vi "Check if good target.vi"(6 "Avg Factor":i32, 7 "Limits":T1, 8 "y2-R":dbl, 9 "x2-R":dbl, 10 "y1-L":dbl, 11 "x1-L":dbl) -> (0 "y2 (R) out":dbl, 1 "x2 (L) out":dbl, 2 "y1 (L) out":dbl, 3 "x1 (L) out":dbl, 5 "Good target?":bool)   [LabVIEW 2018]
uses:
  <vilib>/ptbypt/NI_PtbyPt.lvlib
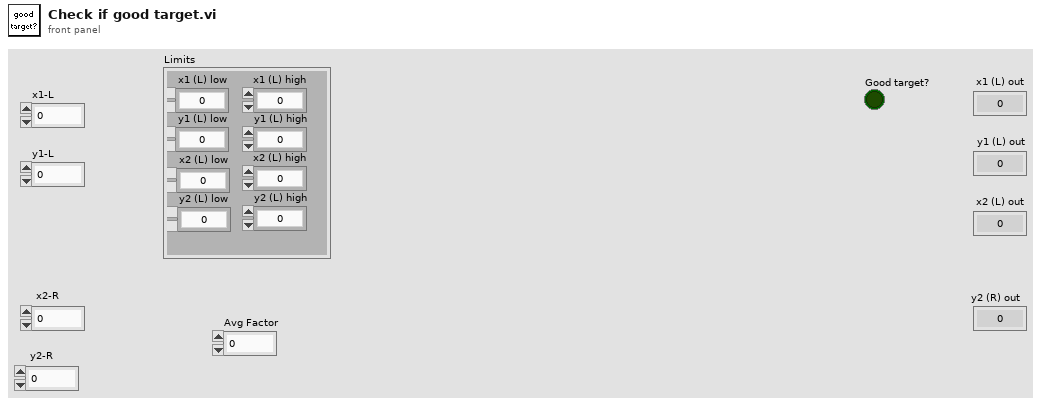
[diagram p1: front panel]
types:
  T1 = cluster{"x1 (L) low":dbl, "x1 (L) high":dbl, "y1 (L) low ":dbl, "y1 (L) high":dbl, "x2 (L) low":dbl, "x2 (L) high":dbl, "y2 (L) low":dbl, "y2 (L) high":dbl}
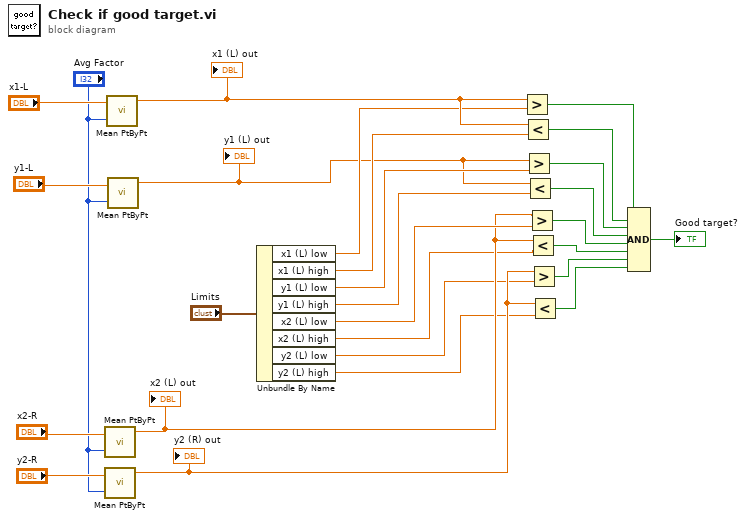
[diagram p0: block diagram]
diagram:
  n1 = call <vilib>:"Mean PtByPt.vi"("x"="x2-R", "sample length"="Avg Factor") -> ("mean"=w14:dbl)  [unwired: 2 in, 1 out]
  "x2 (L) out" <- w14
  n2 = call <vilib>:"Mean PtByPt.vi"("x"="y2-R", "sample length"="Avg Factor") -> ("mean"=w12:dbl)  [unwired: 2 in, 1 out]
  "y2 (R) out" <- w12
  n3 = call <vilib>:"Mean PtByPt.vi"("x"="x1-L", "sample length"="Avg Factor") -> ("mean"=w22:dbl)  [unwired: 2 in, 1 out]
  "x1 (L) out" <- w22
  n4 = call <vilib>:"Mean PtByPt.vi"("x"="y1-L", "sample length"="Avg Factor") -> ("mean"=w17:dbl)  [unwired: 2 in, 1 out]
  "y1 (L) out" <- w17
  n5 = Unbundle By Name("Limits") -> ("x1 (L) low"=w20:dbl, "x1 (L) high"=w19:dbl, "y1 (L) low"=w18:dbl, "y1 (L) high"=w16:dbl, "x2 (L) low"=w15:dbl, "x2 (L) high"=w13:dbl, "y2 (L) low"=w11:dbl, "y2 (L) high"=w10:dbl)
  n6 = Greater?(x=w22, y=w20) -> (0:w9:bool)
  n7 = Less?(x=w22, y=w19) -> (x < y?=w8:bool)
  n8 = Greater?(x=w17, y=w18) -> (0:w7:bool)
  n9 = Less?(x=w17, y=w16) -> (x < y?=w6:bool)
  n10 = Greater?(x=w14, y=w15) -> (0:w5:bool)
  n11 = Less?(x=w14, y=w13) -> (x < y?=w4:bool)
  n12 = Greater?(x=w12, y=w11) -> (0:w3:bool)
  n13 = Less?(x=w12, y=w10) -> (x < y?=w2:bool)
  n14 = Compound Arithmetic op=AND(w9, w8, w7, w6, w5, w4, w3, w2) -> (→"Good target?":bool)
